vi "gen_res_segment.vi"(9 "resonant trigger":bool, 10 "counter cluster in":T1, 11 "scan specification":T2={"x amplitude"=0, "x resolution (pixels)"=0, "x offset fly-forward (iterations)"=0, "x offset fly-back (iterations)"=0, "y resolution (nr. of lines)"=0, "y step size"=0, "iterations per pixel"=0, "number of frames"=0, "y offset (pixels)"=0, "number of y-brake lines  (before y-fly-back)"=0, "number y-brake lines (after y-fly-back)"=0, "number of y-fly-back steps"=8, "lines per z step"=0, "number of z/intensity tuples"=0, "number of repetitions (volumes or planes)"=0}) -> (2 "in recording segment?":bool, 3 "counter cluster out":T1)   [LabVIEW 2010]
uses:
  counter_cluster.ctl
  scan_specification_cluster.ctl
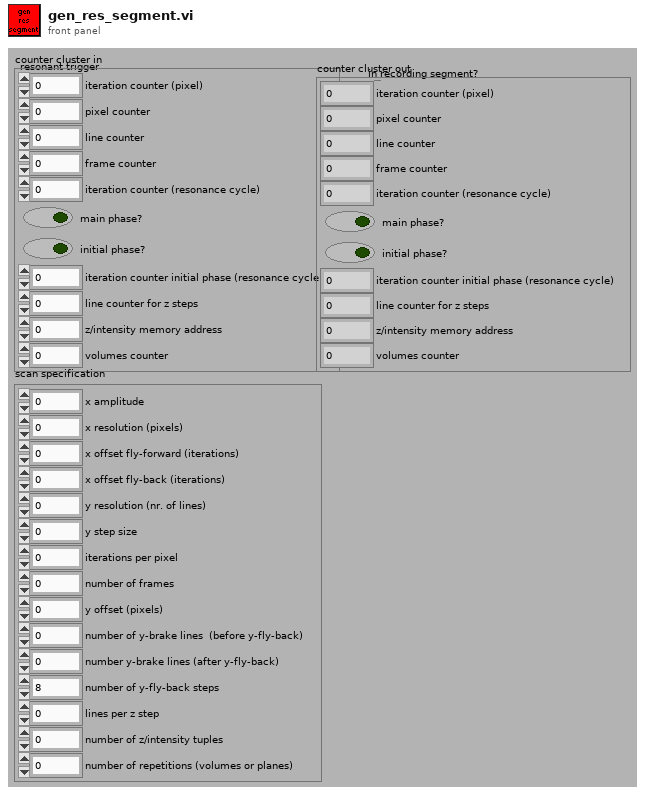
[diagram p1: front panel]
types:
  T1 = typedef "counter_cluster.ctl" = cluster{"iteration counter (pixel)":u16, "pixel counter":u16, "line counter":u16, "frame counter":u16, "iteration counter (resonance cycle)":u16, "main phase?":bool, "initial phase?":bool, "iteration counter initial phase (resonance cycle)":u16, "line counter for z steps":u16, "z/intensity memory address":u32, "volumes counter":u16}
  T2 = typedef "scan_specification_cluster.ctl" = cluster{"x amplitude":u16, "x resolution (pixels)":u16, "x offset fly-forward (iterations)":u16, "x offset fly-back (iterations)":u16, "y resolution (nr. of lines)":u16, "y step size":u16, "iterations per pixel":u16, "number of frames":i32, "y offset (pixels)":u16, "number of y-brake lines  (before y-fly-back)":u16, "number y-brake lines (after y-fly-back)":u16, "number of y-fly-back steps":u16, "lines per z step":u16, "number of z/intensity tuples":u16, "number of repetitions (volumes or planes)":i32}
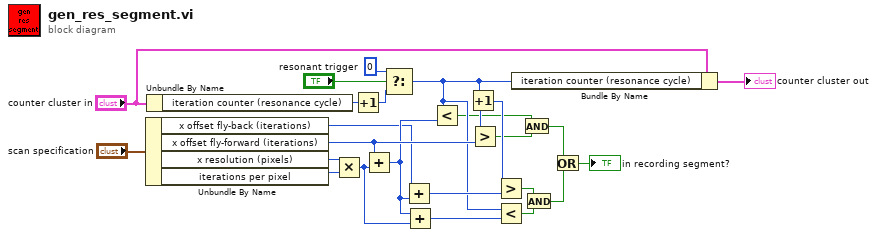
[diagram p0: block diagram]
diagram:
  n1 = Unbundle By Name("scan specification") -> ("x offset fly-back (iterations)"=w4:u16, "x offset fly-forward (iterations)"=w23:u16, "x resolution (pixels)"=w7:u16, "iterations per pixel"=w6:u16)
  n2 = Unbundle By Name("counter cluster in") -> ("iteration counter (resonance cycle)"=w10:u16)
  n3 = Multiply(x=w7, y=w6) -> (x*y=w19:u16)
  n4 = Increment(x=w10) -> (x+1=w9:u16)
  n5 = Add(x=w23, y=w19) -> (x+y=w5:u16)
  n6 = Select(t=u16 0 ("f"), s="resonant trigger", f=w9) -> (s? t:f=w11:u16)
  n7 = Add(x=w4, y=w5) -> (x+y=w20:u16)
  n8 = Add(x=w5, y=w19) -> (x+y=w18:u16)
  n9 = Less?(x=w11, y=w5) -> (x < y?=w2:bool)
  n10 = Increment(x=w11) -> (x+1=w21:u16)
  n11 = Greater?(x=w21, y=w23) -> (0:w3:bool)
  n12 = Greater?(x=w21, y=w20) -> (0:w17:bool)
  n13 = Less?(x=w11, y=w18) -> (x < y?=w16:bool)
  n14 = Bundle By Name(cluster="counter cluster in", "iteration counter (resonance cycle)"=w11) -> (→"counter cluster out":T1)
  n15 = And(x=w2, y=w3) -> (x .and. y?=w22:bool)
  n16 = And(x=w17, y=w16) -> (x .and. y?=w15:bool)
  n17 = Or(x=w22, y=w15) -> (x .or. y?=→"in recording segment?":bool)
